vi "Paste Gray Image.vi"(4 "Height Map":T1, 6 "Focused Image":T1, 8 "error in (no error)":errorcluster, 10 "Max Image Stack":T1[](array[typedef]), 11 "Image Stack":T1[](array[typedef])) -> (0 "error out":errorcluster, 2 "Height Map":T1(plugin-control), 3 "Focused Image":T1(plugin-control))   [LabVIEW 2013]
uses:
  <vilib>/vision/Image Controls.llb/IMAQ Image.ctl
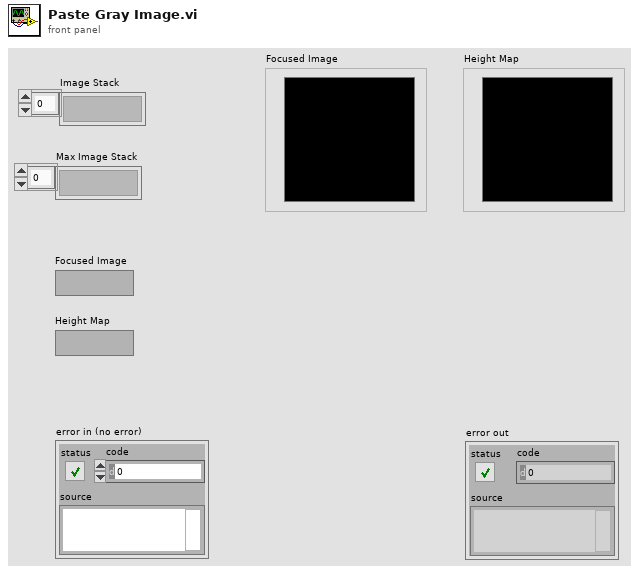
[diagram p1: front panel]
types:
  T1 = typedef "IMAQ Image.ctl" = refnum<image>
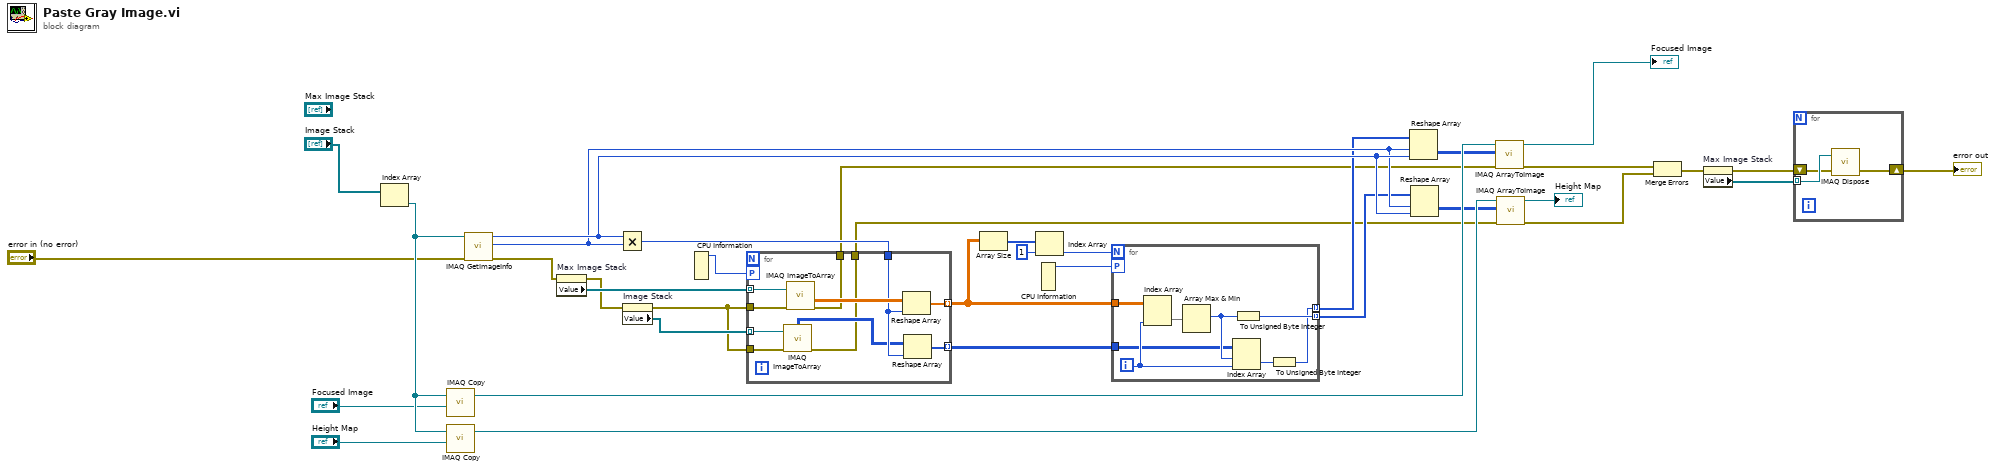
[diagram p0: block diagram]
diagram:
  n1 = Index Array(array="Image Stack") -> (element=w12:T1)  [unwired: 1 in]
  n2 = call "IMAQ Copy"("Image Dst"="Focused Image", "Image Src"=w12) -> ("Image Dst Out"=w29:T1)  [unwired: 4 in, 1 out]
  n3 = call "IMAQ Copy"("Image Dst"="Height Map", "Image Src"=w12) -> ("Image Dst Out"=w30:T1)  [unwired: 4 in, 1 out]
  n4 = call "IMAQ GetImageInfo"("error in (no error)"="error in (no error)", "Image"=w12) -> ("error out"=w36:errorcluster, "Y Resolution"=w34:i32, "X Resolution"=w35:i32)  [unwired: 2 in, 5 out]
  n5 = property on="Max Image Stack" class="Arr (strict)"(error in=w36) -> (error out=w16:errorcluster, "Value"=w25:T1[])  [unwired: 1 in, 1 out]
  n6 = Multiply(x=w35, y=w34) -> (x*y=w24:i32)
  n7 = property on="Image Stack" class="Arr (strict)"(error in=w16) -> (error out=w11:errorcluster, "Value"=w15:T1[])  [unwired: 1 in, 1 out]
  n8 = CPU Information() -> (4:w5:i32)  [unwired: 3 out]
  n9 = for {
    tunnel: w25 -> [w47] mode=indexing
    tunnel: w24 -> [w43]
    tunnel: [w45] -> w21 mode=indexing
    tunnel: w11 -> [w44]
    workers-P: w5 -> [_]
    tunnel: [w42] -> w14 mode=indexing
    tunnel: w15 -> [w41] mode=indexing
    tunnel: w11 -> [w39]
    tunnel: [w38] -> w8
    tunnel: [w37] -> w7
    n10 = call "IMAQ ImageToArray"("error in (no error)"=w39, "Image"=w41) -> ("error out"=w37:errorcluster, "Image Pixels (U8)"=w40:u8[][])  [unwired: 2 in, 3 out]
    n11 = call "IMAQ ImageToArray"("error in (no error)"=w44, "Image"=w47) -> ("Image Pixels (Float)"=w46:sgl[][], "error out"=w38:errorcluster)  [unwired: 2 in, 3 out]
    n12 = Reshape Array(w46, w43) -> (w45:sgl[])
    n13 = Reshape Array(w40, w43) -> (w42:u8[])
  }
  n14 = Array Size(array=w21) -> (size(s)=w23:i32[])
  n15 = CPU Information() -> (4:w4:i32)  [unwired: 3 out]
  n16 = Index Array(array=w23, index=1) -> (element=w22:i32)
  n17 = for {
    N: w22 -> [_]
    tunnel: w21 -> [w55]
    tunnel: [w48] -> w17 mode=indexing
    tunnel: [w53] -> w19 mode=indexing
    tunnel: w14 -> [w50]
    workers-P: w4 -> [_]
    i -> [w52]
    n18 = Index Array(array=w55, index (col)=w52) -> (element=w54:sgl[])  [unwired: 1 in]
    n19 = Array Max & Min(array=w54) -> (max index (indices)=w51:i32)  [unwired: 3 out]
    n20 = Index Array(array=w50, index (row)=w51, index (col)=w52) -> (element=w49:u8)
    n21 = To Unsigned Byte Integer(number=w51) -> (unsigned 8bit integer=w53:u8)
    n22 = To Unsigned Byte Integer(number=w49) -> (unsigned 8bit integer=w48:u8)
  }
  n23 = Reshape Array(w17, w34, w35) -> (w13:u8[][])
  n24 = Reshape Array(w19, w34, w35) -> (w18:u8[][])
  n25 = call "IMAQ ArrayToImage"("error in (no error)"=w8, "Image Pixels (U8)"=w13, "Image"=w29) -> ("error out"=w10:errorcluster, "Image Out"=→"Focused Image":T1)  [unwired: 7 in]
  n26 = call "IMAQ ArrayToImage"("error in (no error)"=w7, "Image Pixels (U8)"=w18, "Image"=w30) -> ("error out"=w9:errorcluster, "Image Out"=→"Height Map":T1)  [unwired: 7 in]
  n27 = Merge Errors(w10, w9) -> (w6:errorcluster)
  n28 = property on="Max Image Stack" class="Arr (strict)"(error in=w6) -> (error out=w31:errorcluster, "Value"=w33:T1[])  [unwired: 1 in, 1 out]
  n29 = for {
    tunnel: w33 -> [w58] mode=indexing
    shift-right: [w57] -> w32
    shift-left: w31 -> [w56]
    n30 = call "IMAQ Dispose"("Image"=w58, "error in (no error)"=w56) -> ("error out"=w57:errorcluster)  [unwired: 4 in]
  }
  "error out" <- w32
